vi "re-initiate.vi"(0 "reference in":refnum<class "Notification Controller.lvclass">, 5 "error in (no error)":errorcluster) -> (14 "reference out":refnum<class "Notification Controller.lvclass">, 19 "error out":errorcluster)   [LabVIEW 2016, in "Notification Controller.lvclass"]
uses:
  Notification Controller.lvclass
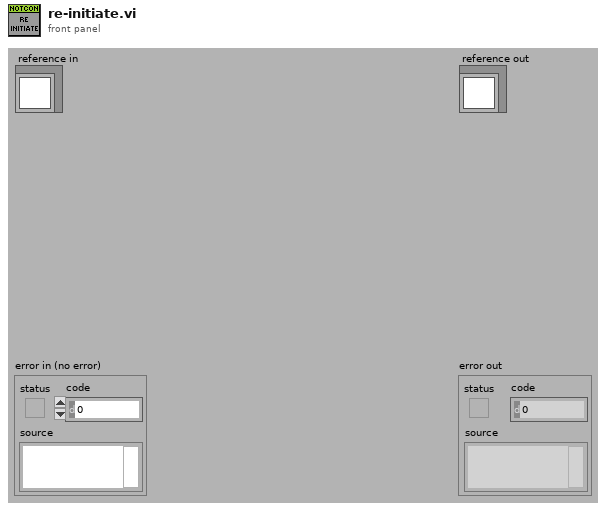
[diagram p1: front panel]
types:
  T1 = typedef "Notification Controller.lvclass/ObjectAttributesRef.ctl" = refnum<data-value>
  T2 = typedef "Notification Controller.lvclass/ObjectAttributes.ctl" = cluster{"MyAttribute":dbl, "items_data":string[][][], "items_notification_refs":refnum<class "itemsNotification.lvclass">[], "notifications_data_items":string[][], "items_nots?":bool, "devices_controller_ref":refnum<class "Devices Controller.lvclass">, "onlineUpdate":timestamp, "notController?":bool, "tracking_notification_ref":refnum<class "trackingNotification.lvclass">, "notifications_data_tracking":string[][], "tracking_parts_data":string[][], "tracking_nots?":bool, "index_tracking_not":i32[], "file_controller_ref":refnum<class "File Controller.lvclass">}
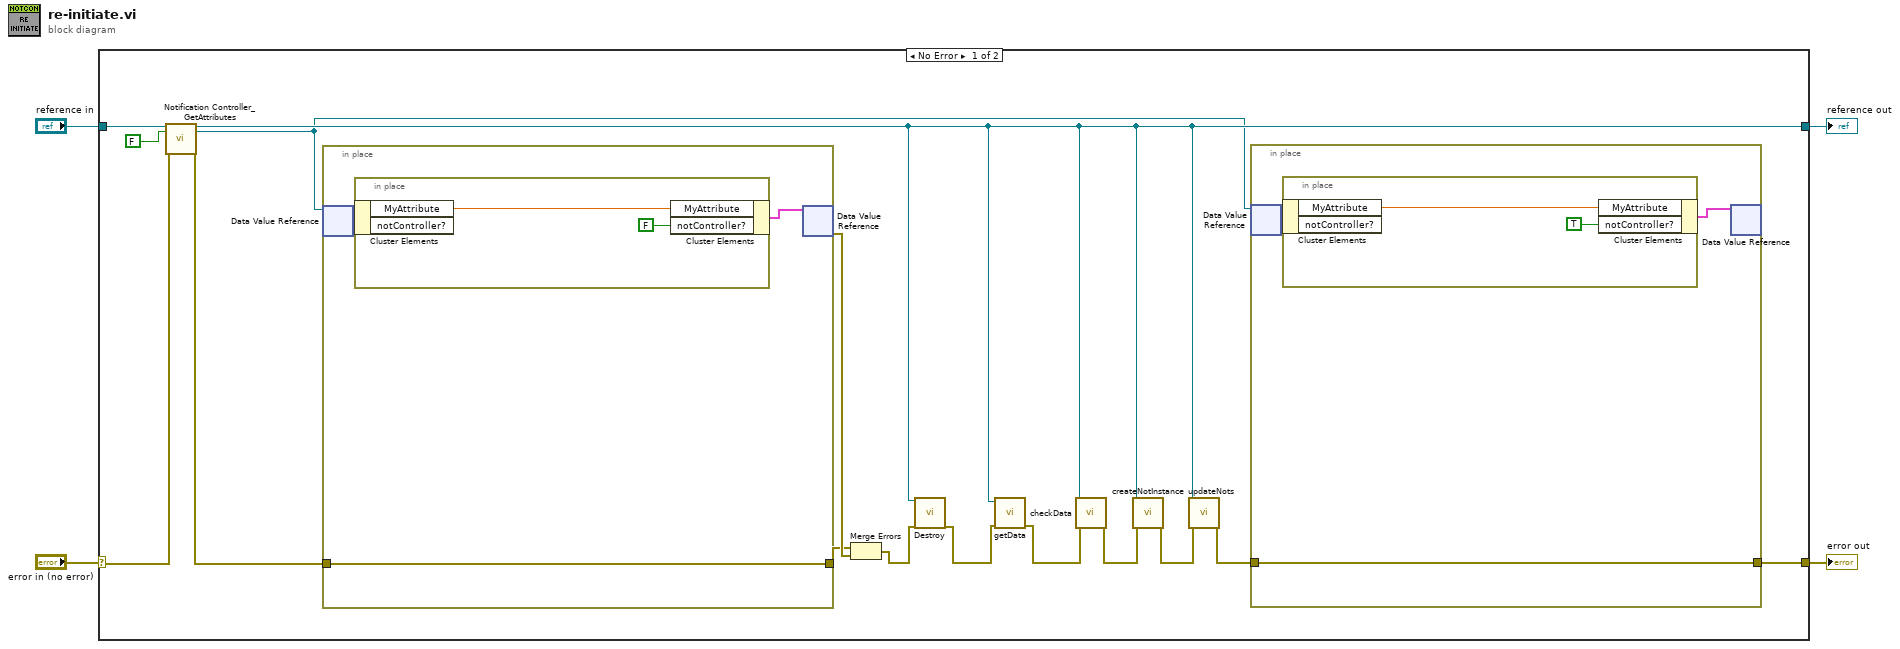
[diagram p0: block diagram]
diagram:
  n1 = case shown="No Error" "error in (no error)" {
    selector: "error in (no error)" -> [w15 w31]
    tunnel: [w6 w31] -> w3
    tunnel: [w8 w30] -> w1
    tunnel: "reference in" -> [w17 w30]
    frame No Error {
      n2 = call "Notification Controller_GetAttributes.vi"("reference in"=w17, "return data? (T)"=FALSE, "error in (no error)"=w15) -> ("reference out"=w8:refnum<class "Notification Controller.lvclass">, "attributes ref"=w5:T1, "error out"=w12:errorcluster)  [unwired: 13 in, 1 out]
      n3 = in-place {
        in-place-border: w12 -> [w25]
        in-place-border: [w25] -> w18
        n4 = in-place-dvr #1(w5) -> (w26:T2)  [unwired: 1 out]
        n5 = in-place {
          n6 = in-place-cluster #2(w26) -> ("MyAttribute"=w29:dbl)  [unwired: 1 out]
          n7 = in-place-cluster #2("MyAttribute"=w29, "notController?"=FALSE) -> (w27:T2)
        }
        n8 = in-place-dvr #1(w27) -> (w19:errorcluster)  [unwired: 1 out]
      }
      n9 = Merge Errors(w18, w19) -> (w11:errorcluster)
      n10 = call-dynamic "Destroy.vi"("reference in"=w8, "error in (no error)"=w11) -> ("error out"=w10:errorcluster)  [unwired: 16 in, 1 out]
      n11 = call "getData.vi"("error in (no error)"=w10, "reference in"=w8) -> ("error out"=w9:errorcluster)  [unwired: 7 in, 2 out]
      n12 = call "checkData.vi"("error in (no error)"=w9, "reference in"=w8) -> ("error out"=w14:errorcluster)  [unwired: 8 in, 1 out]
      n13 = call "createNotInstance.vi"("error in (no error)"=w14, "reference in"=w8) -> ("error out"=w13:errorcluster)  [unwired: 8 in, 1 out]
      n14 = call "updateNots.vi"("error in (no error)"=w13, "reference in"=w8) -> ("error out"=w7:errorcluster)  [unwired: 8 in, 1 out]
      n15 = in-place {
        in-place-border: w7 -> [w20]
        in-place-border: [w20] -> w6
        n16 = in-place-dvr #3(w5) -> (w21:T2)  [unwired: 1 out]
        n17 = in-place {
          n18 = in-place-cluster #4(w21) -> ("MyAttribute"=w24:dbl)  [unwired: 1 out]
          n19 = in-place-cluster #4("MyAttribute"=w24, "notController?"=TRUE) -> (w22:T2)
        }
        n20 = in-place-dvr #3(w22) -> ()  [unwired: 2 out]
      }
    }
    frame Error {
    }
  }
  "error out" <- w3
  "reference out" <- w1
